vi "CalculateTotalIonEnergy.vi"(9 "Ion Charge State":u8, 10 "Total Source Ion Energy (kV)":dbl, 11 "Terminal Voltage (V)":dbl) -> (3 "Total Ion Energy (MeV)":dbl)   [LabVIEW 2012]
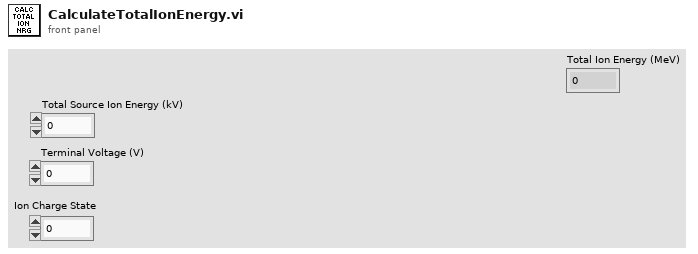
[diagram p1: front panel]
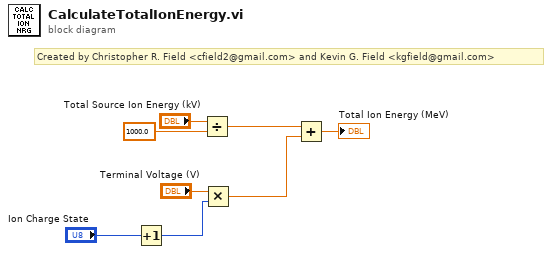
[diagram p0: block diagram]
diagram:
  # "Created by Christopher R. Field <cfield2@gmail.com> and Kevin G. Field <kgfield@gmail.com>"
  n1 = Increment(x="Ion Charge State") -> (x+1=w5:u8)
  n2 = Divide(x="Total Source Ion Energy (kV)", y=1000.0) -> (x/y=w7:dbl)
  n3 = Multiply(x="Terminal Voltage (V)", y=w5) -> (x*y=w4:dbl)
  n4 = Add(x=w7, y=w4) -> (x+y=→"Total Ion Energy (MeV)":dbl)
